vi "PDF Details wit Doc.vi"(0 "PDF Document IN":refnum<k24>, 7 "PDF Details":T1, 11 "error in (no error)":errorcluster) -> (4 "PDF Document OUT":refnum<k24>, 15 "error out":errorcluster)   [LabVIEW 2019, in "Exaprom PDF.lvlib"]
doc: "Write some metadatas to the PDF file:\n- Title\n- Subject\n- Keyword\n- Author\n- Creator\n\nVersion 1.0\nDeveloped by Jean-Marc Simard\nCopyright © 2010, Exaprom Inc.\nAll rights reserved.\nLicense: BSD\n\nWith iTextSharp 4.1.6 (http://itextsharp.sourceforge.net)\nunder Mozilla Public License Version 1.1\n(http://www.mozilla.org/MPL/MPL-1.1.html)"
uses:
  Controls/Initialization Controls/PDF Details.ctl
  C:/work/niobrara_lv/labview pdf writer fixing/DLL/itextsharp.dll
  DLL/itextsharp.dll
  Exaprom PDF.lvlib
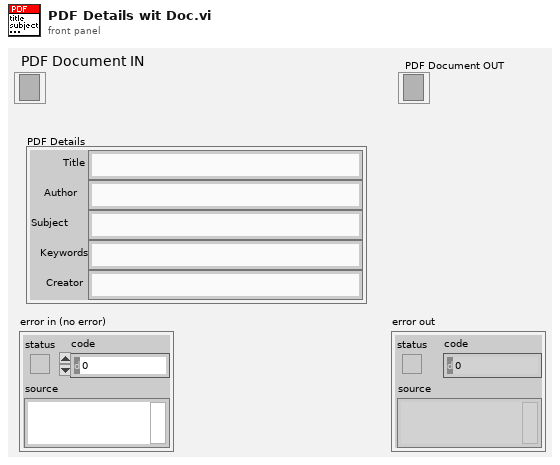
[diagram p1: front panel]
types:
  T1 = typedef "Exaprom PDF.lvlib/PDF Details.ctl" = cluster{"Title":string, "Author":string, "Subject":string, "Keywords":string, "Creator":string}
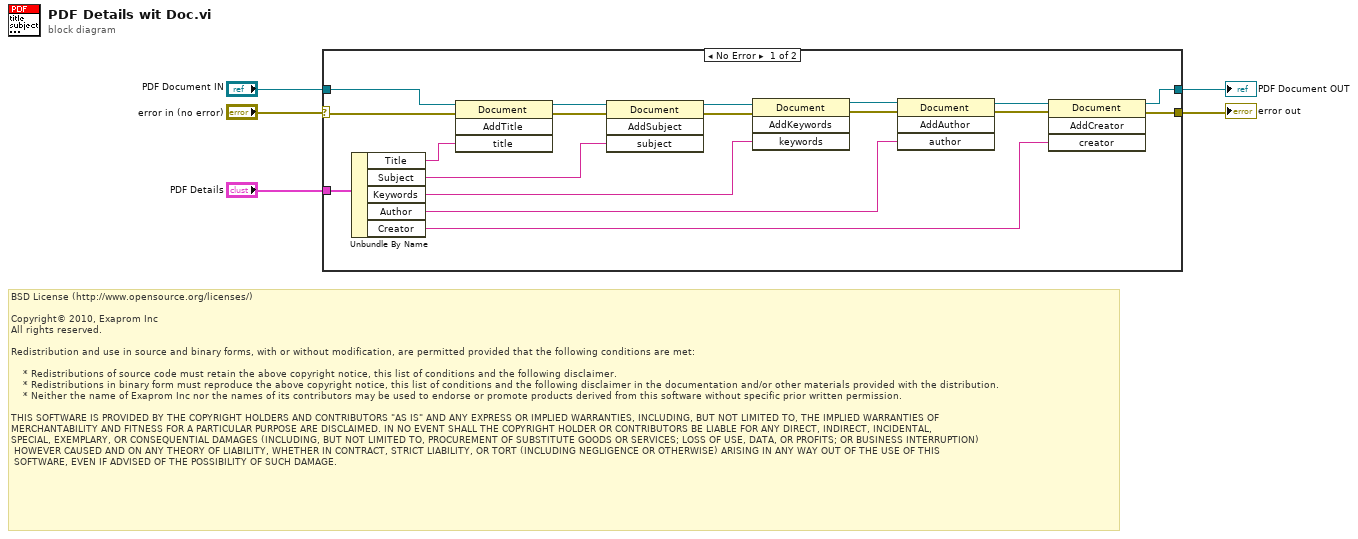
[diagram p0: block diagram]
diagram:
  # "BSD License (http://www.opensource.org/licenses/)\n\nCopyright© 2010, Exaprom Inc\nAll rights reserved.\n\nRedistribution and use in source and binary forms, with or without modification, are permitted provided that the following conditions are met:\n\n    * Redistributions of source code must retain the above copyright notice, this list of conditions and the following disclaimer.\n    * Redistributions in binary form must reproduce the above copyright notice, this list of conditions and the following disclaimer in the documentation and/or other materials provided with the distribution.\n    * Neither the name of Exaprom Inc nor the names of its contributors may be used to endorse or promote products derived from this software without specific prior written permission.\n\nTHIS SOFTWARE IS PROVIDED BY THE COPYRIGHT HOLDERS AND CONTRIBUTORS \"AS IS\" AND ANY EXPRESS OR IMPLIED WARRANTIES, INCLUDING, BUT NOT LIMITED TO, THE IMPLIED WARRANTIES OF \nMERCHANTABILITY AND FITNESS FOR A PARTICULAR PURPOSE ARE DISCLAIMED. IN NO EVENT SHALL THE COPYRIGHT HOLDER OR CONTRIBUTORS BE LIABLE FOR ANY DIRECT, INDIRECT, INCIDENTAL,\nSPECIAL, EXEMPLARY, OR CONSEQUENTIAL DAMAGES (INCLUDING, BUT NOT LIMITED TO, PROCUREMENT OF SUBSTITUTE GOODS OR SERVICES; LOSS OF USE, DATA, OR PROFITS; OR BUSINESS INTERRUPTION)\n HOWEVER CAUSED AND ON ANY THEORY OF LIABILITY, WHETHER IN CONTRACT, STRICT LIABILITY, OR TORT (INCLUDING NEGLIGENCE OR OTHERWISE) ARISING IN ANY WAY OUT OF THE USE OF THIS\n SOFTWARE, EVEN IF ADVISED OF THE POSSIBILITY OF SUCH DAMAGE."
  n1 = case shown="No Error" "error in (no error)" {
    selector: "error in (no error)" -> [w7 w25]
    tunnel: "PDF Details" -> [w23 _]
    tunnel: [w14 w25] -> w4
    tunnel: "PDF Document IN" -> [w6 w24]
    tunnel: [w8 w24] -> w2
    frame No Error {
      n2 = Unbundle By Name(w23) -> ("Title"=w9:string, "Subject"=w13:string, "Keywords"=w12:string, "Author"=w11:string, "Creator"=w10:string)
      n3 = invoke class="Document" method="AddTitle"(reference=w6, error in=w7, "title"=w9) -> (reference out=w22:refnum<k24>, error out=w21:errorcluster)  [unwired: 1 in, 2 out]
      n4 = invoke class="Document" method="AddSubject"(reference=w22, error in=w21, "subject"=w13) -> (reference out=w20:refnum<k24>, error out=w19:errorcluster)  [unwired: 1 in, 2 out]
      n5 = invoke class="Document" method="AddKeywords"(reference=w20, error in=w19, "keywords"=w12) -> (reference out=w18:refnum<k24>, error out=w17:errorcluster)  [unwired: 1 in, 2 out]
      n6 = invoke class="Document" method="AddAuthor"(reference=w18, error in=w17, "author"=w11) -> (reference out=w15:refnum<k24>, error out=w16:errorcluster)  [unwired: 1 in, 2 out]
      n7 = invoke class="Document" method="AddCreator"(reference=w15, error in=w16, "creator"=w10) -> (reference out=w8:refnum<k24>, error out=w14:errorcluster)  [unwired: 1 in, 2 out]
    }
    frame Error {
    }
  }
  "error out" <- w4
  "PDF Document OUT" <- w2
